vi "Stop Core.vi"(10 "final error code":i32, 11 "CameraTestingENI":refnum<class "CameraTestingENI.lvclass">) -> (3 "CameraTestingENI":refnum<class "CameraTestingENI.lvclass">)   [LabVIEW 2020, in "CameraTestingProxy.lvlib" / "CameraTestingENI.lvclass"]
doc: "(<B>Filename</B>: Actor Framework.lvlib:Actor.lvclass:Stop Core.vi)\n\nDefines what the actor does before it stops. Use the <B>final error code</B> input to determine whether the actor shut down in response to an error.\n\nBy default, this method passes the Stop message along to all auto-stop nested actors. A descendant class may override this method to define additional behavior, such as shutting down any processes the actor initiated in its override of the Actor Core method."
uses:
  CameraTestingENI.lvclass
  CameraTestingENI.lvclass/CameraTestingENI.ctl
  <vilib>/ActorFramework/Actor/Actor.lvclass
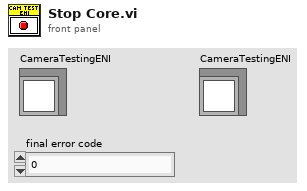
[diagram p1: front panel]
types:
  T1 = typedef "CameraTestingProxy.lvlib/CameraTestingENI.lvclass/QuitActorEvn.ctl" = refnum<user-event>
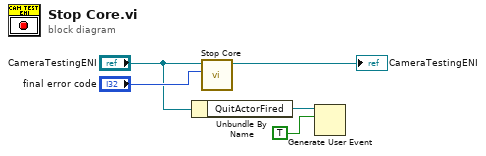
[diagram p0: block diagram]
diagram:
  n1 = Unbundle By Name("CameraTestingENI") -> ("QuitActorFired"=w2:T1)
  n2 = call-parent "Stop Core.vi"("final error code"="final error code", "Actor in"="CameraTestingENI") -> ("Actor out"=→"CameraTestingENI":refnum<class "CameraTestingENI.lvclass">)  [unwired: 9 in]
  n3 = Generate User Event(user event=w2, event data cluster=TRUE ("event data")) -> ()  [unwired: 2 in, 2 out]
